vi "New from Folder (Factory).vi"(7 "Logger":refnum<class "Logger.lvclass">, 8 "error in (no error)":errorcluster, 9 "Name (Auto)":string, 10 "Folder":path) -> (0 "error out":errorcluster, 3 "PackageAbstract out":refnum<class "PackageAbstract.lvclass">)   [LabVIEW 2020, in "GPack.lvlib" / "PackageAbstract.lvclass"]
uses:
  PackageAbstract.lvclass
  Logger/Logger.lvclass
  GPack.lvlib
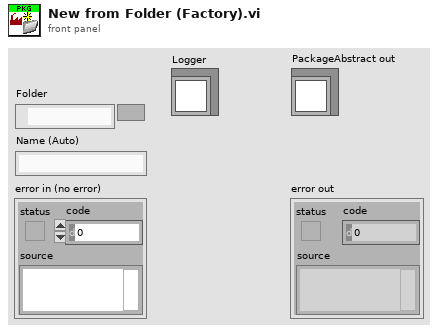
[diagram p1: front panel]
types:
  T1 = typedef "GPack.lvlib/Package Info.ctl" = cluster{"Name":string, "Type":string, "Host":string, "Path":string, "Branch":string, "Version":string, "License":string}
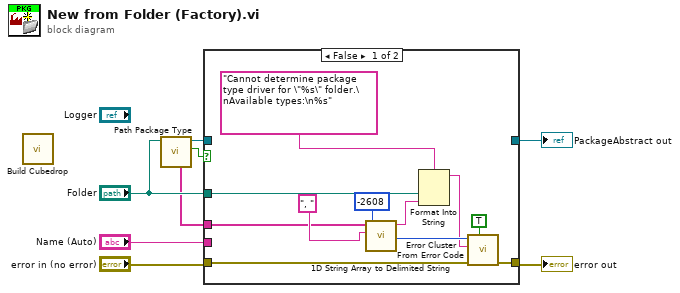
[diagram p0: block diagram]
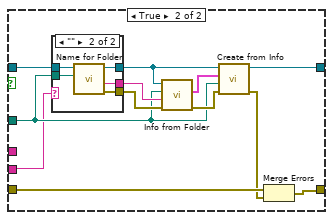
[diagram p2: hidden frame]
diagram:
  n1 = call "Build Cubedrop.vi"() -> ()  [unwired: 12 in]
  n2 = call "Path Package Type.vi"("Path"="Folder") -> ("Matched"=w1:bool, "First Match"=w2:refnum<class "PackageAbstract.lvclass">, "Available Types"=w3:string[])  [unwired: 7 in, 1 out]
  n3 = case shown="False" w1 {
    tunnel: "error in (no error)" -> [w18 w23]
    tunnel: w2 -> [_ w30]
    tunnel: "Folder" -> [w14 w20]
    tunnel: [w16 w21] -> w7
    tunnel: [_ w24] -> w6
    tunnel: w3 -> [w9 _]
    tunnel: "Name (Auto)" -> [_ w19]
    frame False {
      n4 = call <vilib>:"1D String Array to Delimited String.vi"("delimiter"=", ", "string array"=w9) -> ("delimited string"=w12:string)  [unwired: 9 in]
      n5 = Format Into String(format string="Cannot determine package type driver for \"%s\" folder.\nAvailable types:\n%s", w14, w12) -> (resulting string=w10:string)  [unwired: 2 in, 1 out]
      n6 = call <vilib>:"Error Cluster From Error Code.vi"("show call chain? (False)"=TRUE, "error in (no error)"=w18, "error message (\"\")"=w10, "error code (0)"=-2608) -> ("error out"=w16:errorcluster)  [unwired: 5 in]
    }
    frame True {
      n7 = case shown="\"\"" w19 {
        selector: w19 -> [w31 _]
        tunnel: w30 -> [w32 w37]
        tunnel: [w31 w36] -> w29
        tunnel: [_ w35] -> w28
        tunnel: [w32 w34] -> w25
        tunnel: w20 -> [_ w33]
        frame Default {
        }
        frame "" {
          n8 = call "Name for Folder.vi"("Folder"=w33, "PackageAbstract in"=w37) -> ("error out"=w35:errorcluster, "Name"=w36:string, "PackageAbstract out"=w34:refnum<class "PackageAbstract.lvclass">)  [unwired: 6 in, 1 out]
        }
      }
      n9 = call-dynamic "Info from Folder.vi"("error in (no error)"=w28, "Name"=w29, "Folder"=w20, "Package in"=w25) -> ("error out"=w27:errorcluster, "Package Info"=w26:T1)  [unwired: 6 in]
      n10 = call-dynamic "Create from Info.vi"("error in (no error)"=w27, "Folder"=w20, "Package Info"=w26, "Package in"=w25) -> ("error out"=w22:errorcluster, "Package out"=w24:refnum<class "PackageAbstract.lvclass">)  [unwired: 6 in]
      n11 = Merge Errors(w23, w22) -> (w21:errorcluster)
    }
  }
  "error out" <- w7
  "PackageAbstract out" <- w6
